vi "SmoothPathGenerator.vi"(1 "TargetOrientation":dbl=270.0, 2 "RobotOrientation":dbl=70.0, 3 "DeltaY":dbl=60.0, 4 "DeltaX":dbl=60.0) -> (0 "SmoothPath":cluster{dbl, dbl}[](array[cluster]))   [LabVIEW 2018]
uses:
  Dawgma-Programming-Library-master/Dawgma-Programming-Library-master/Controls/PurePursuit/RobotNeededPathData.ctl
panel:
  in  "TargetPointOffset":dbl=12.0
  in  "RobotPointOffset":dbl=12.0
  out "Smoothed":cluster{dbl[], dbl[]}(graph)
  out "Waypoints":cluster{dbl[], dbl[]}(graph)
  in  "PointInjectionSpacing":dbl=6.0
  in  "Path":cluster{"x":dbl, "y":dbl}[](array[cluster])=[{"x"=0.0, "y"=0.0}, {"x"=0.0, "y"=0.0}, {"x"=0.0, "y"=0.0}, {"x"=0.0, "y"=0.0}, {"x"=0.0, "y"=0.0}]
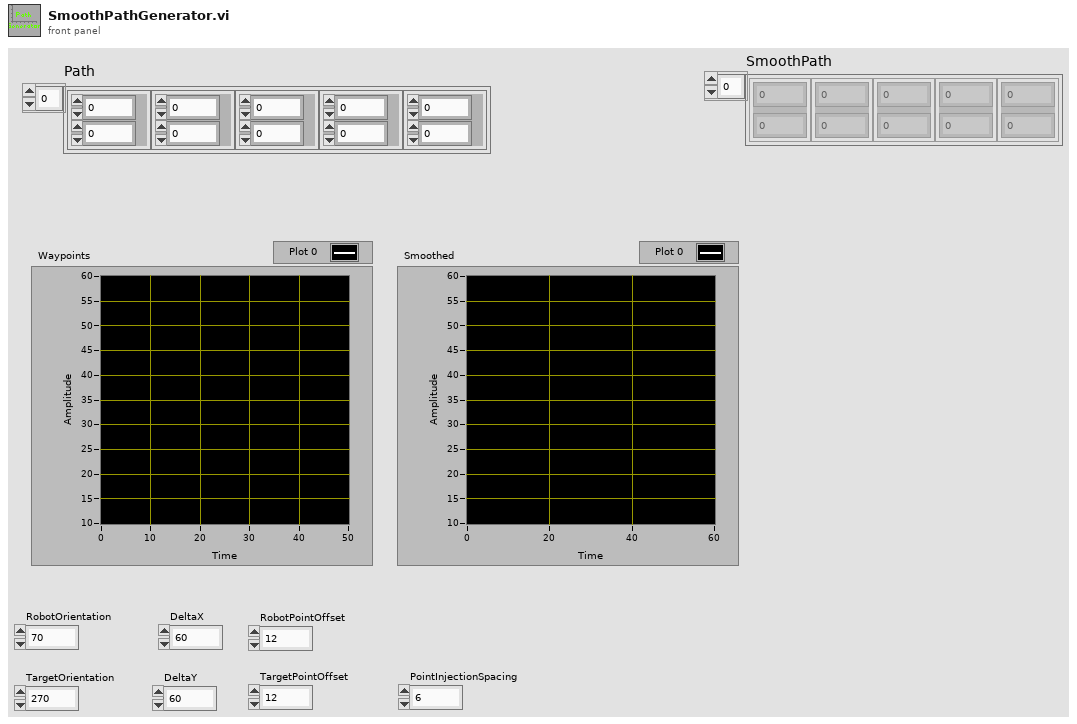
[diagram p1: front panel]
types:
  T1 = typedef "RobotNeededPathData.ctl" = cluster{"Path":cluster{dbl, dbl}[], "MaxVel":dbl, "MaxAccel":dbl, "Backwards?":bool, "PointSpacing":dbl, "LookaheadDist":dbl, "Speed/Curve":dbl, "SlowDistanceAtEnd":dbl, "SlowSpeed":dbl, "MaxDeAccel":dbl}
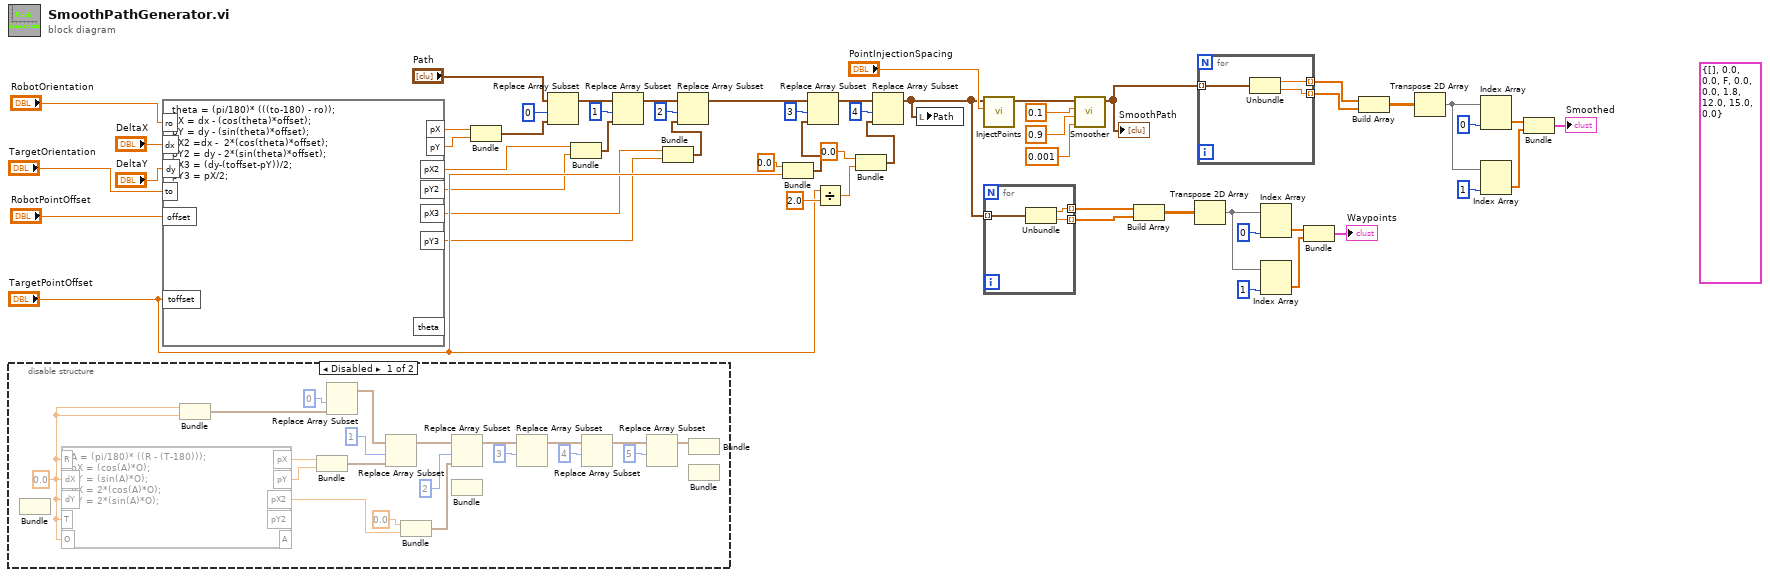
[diagram p0: block diagram]
diagram:
  (unwired) T1 {"Path"=[], "MaxVel"=0.0, "MaxAccel"=0.0, "Backwards?"=FALSE, "PointSpacing"=0.0, "LookaheadDist"=0.0, "Speed/Curve"=1.8, "SlowDistanceAtEnd"=12.0, "SlowSpeed"=15.0, "MaxDeAccel"=0.0} ("RobotNeededPathData")
  n1 = disable-structure shown="Disabled" {
    frame Disabled {
      w60 = 0.0
      n2 = Bundle() -> ()  [unwired: 3 in, 1 out]
      n3 = formula code="A = (pi/180)* ((R - (T-180)));\npX = (cos(A)*O);\npY = (sin(A)*O);\npX = 2*(cos(A)*O);\npY = 2*(sin(A)*O);"("R"=w60, "dX"=w60, "dY"=w60, "T"=w60, "O"=w60) -> ("pX"=w61:dbl, "pY"=w62:dbl, "pX2"=w58:dbl)  [unwired: 2 out]
      n4 = Bundle(w60, w60) -> (w75:cluster{dbl, dbl})  [unwired: 1 in]
      n5 = Bundle("pX"=w61, "pY"=w62) -> (w76:cluster{"pX":dbl, "pY":dbl})  [unwired: 1 in]
      n6 = Replace Array Subset(new element=w75, index=0) -> (w67:cluster{dbl, dbl}[])  [unwired: 1 in]
      n7 = Replace Array Subset(array=w67, new element=w76, index=1) -> (w66:cluster{dbl, dbl}[])
      n8 = Bundle(0.0, "pX2"=w58) -> (w72:cluster{dbl, "pX2":dbl})  [unwired: 1 in]
      n9 = Replace Array Subset(array=w66, new element=w72, index=2) -> (w65:cluster{dbl, dbl}[])
      n10 = Bundle() -> ()  [unwired: 3 in, 1 out]
      n11 = Replace Array Subset(array=w65, index=3) -> (w64:cluster{dbl, dbl}[])  [unwired: 1 in]
      n12 = Replace Array Subset(array=w64, index=4) -> (w63:cluster{dbl, dbl}[])  [unwired: 1 in]
      n13 = Replace Array Subset(array=w63, index=5) -> (w57:cluster{dbl, dbl}[])  [unwired: 1 in]
      n14 = Bundle(w57) -> ()  [unwired: 2 in, 1 out]
      n15 = Bundle() -> ()  [unwired: 3 in, 1 out]
    }
    frame Enabled {
    }
  }
  n16 = formula code="theta = (pi/180)* (((to-180) - ro));\npX = dx - (cos(theta)*offset);\npY = dy - (sin(theta)*offset);\npX2 =dx -  2*(cos(theta)*offset);\npY2 = dy - 2*(sin(theta)*offset);\npX3 = (dy-(toffset-pY))/2;\npY3 = pX/2;"("ro"="RobotOrientation", "dx"="DeltaX", "dy"="DeltaY", "to"="TargetOrientation", "offset"="RobotPointOffset", "toffset"="TargetPointOffset") -> ("pX"=w26:dbl, "pY"=w25:dbl, "pX2"=w7:dbl, "pY2"=w6:dbl, "pX3"=w4:dbl, "pY3"=w3:dbl)  [unwired: 1 out]
  n17 = Bundle("pX"=w26, "pY"=w25) -> (w32:cluster{"pX":dbl, "pY":dbl})  [unwired: 1 in]
  n18 = Replace Array Subset(array="Path", new element=w32, index=0) -> (w33:cluster{"x":dbl, "y":dbl}[])
  n19 = Bundle("pX2"=w7, "pY2"=w6) -> (w5:cluster{"pX2":dbl, "pY2":dbl})  [unwired: 1 in]
  n20 = Replace Array Subset(array=w33, new element=w5, index=1) -> (w23:cluster{"x":dbl, "y":dbl}[])
  n21 = Bundle("pX3"=w4, "pY3"=w3) -> (w2:cluster{"pX3":dbl, "pY3":dbl})  [unwired: 1 in]
  n22 = Replace Array Subset(array=w23, new element=w2, index=2) -> (w1:cluster{"x":dbl, "y":dbl}[])
  n23 = Bundle(0.0, "TargetPointOffset"="TargetPointOffset") -> (w9:cluster{dbl, "TargetPointOffset":dbl})  [unwired: 1 in]
  n24 = Replace Array Subset(array=w1, new element=w9, index=3) -> (w17:cluster{"x":dbl, "y":dbl}[])
  n25 = Divide(x="TargetPointOffset", y=2.0) -> (x/y=w14:dbl)
  n26 = Bundle(0.0, w14) -> (w13:cluster{dbl, dbl})  [unwired: 1 in]
  n27 = Replace Array Subset(array=w17, new element=w13, index=4) -> (w16:cluster{"x":dbl, "y":dbl}[])
  n28 = local write "Path"(w16) -> ()
  n29 = call "InjectPoints.vi"("Spacing"="PointInjectionSpacing", "Path"=w16) -> ("Path out"=w38:cluster{dbl, dbl}[])  [unwired: 9 in]
  n30 = for {
    tunnel: w16 -> [w79] mode=indexing
    tunnel: [w78] -> w55 mode=indexing
    tunnel: [w77] -> w54 mode=indexing
    n31 = Unbundle(w79) -> ("x"=w78:dbl, "y"=w77:dbl)
  }
  n32 = call "Smoother.vi"("tolerance"=0.001, "B"=0.9, "A"=0.1, "Path"=w38) -> ("SmoothPath"=w37:cluster{dbl, dbl}[])  [unwired: 7 in]
  "SmoothPath" <- w37
  n33 = Build Array(w55, w54) -> (w53:dbl[][])
  n34 = Transpose 2D Array(2D array=w53) -> (transposed array=w50:dbl[][])
  n35 = for {
    tunnel: w37 -> [w82] mode=indexing
    tunnel: [w81] -> w46 mode=indexing
    tunnel: [w80] -> w45 mode=indexing
    n36 = Unbundle(w82) -> (w81:dbl, w80:dbl)
  }
  n37 = Index Array(array=w50, index (col)=0 ("disabled index (col)")) -> (element=w48:dbl[])  [unwired: 1 in]
  n38 = Index Array(array=w50, index (col)=1 ("disabled index (col)")) -> (element=w49:dbl[])  [unwired: 1 in]
  n39 = Bundle(w48, w49) -> (→"Waypoints":cluster{dbl[], dbl[]})  [unwired: 1 in]
  n40 = Build Array(w46, w45) -> (w44:dbl[][])
  n41 = Transpose 2D Array(2D array=w44) -> (transposed array=w41:dbl[][])
  n42 = Index Array(array=w41, index (col)=0 ("disabled index (col)")) -> (element=w39:dbl[])  [unwired: 1 in]
  n43 = Index Array(array=w41, index (col)=1 ("disabled index (col)")) -> (element=w40:dbl[])  [unwired: 1 in]
  n44 = Bundle(w39, w40) -> (→"Smoothed":cluster{dbl[], dbl[]})  [unwired: 1 in]
